vi "Initialize DAQ Assistant - Digital.vi"(8 "error in":errorcluster, 9 "rate":dbl=1000.0, 10 "number of samples":i32=100, 11 "physical channels":tag) -> (0 "error out":errorcluster, 3 "task out":refnum<k21>)   [LabVIEW 2021]
uses:
  <vilib>/DAQmx/create/channels.llb/DAQmx Create Channel (DI-Digital Input).vi
  <vilib>/DAQmx/configure/timing.llb/DAQmx Timing (Sample Clock).vi
  <resource>/objmgr/daqmx.rc
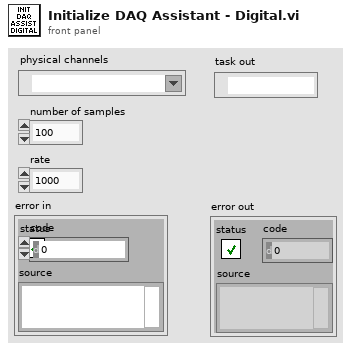
[diagram p1: front panel]
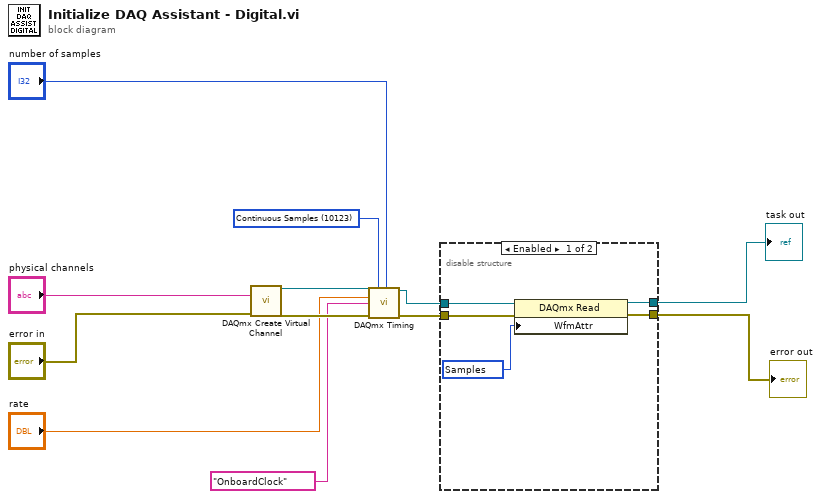
[diagram p0: block diagram]
diagram:
  w10 = 10123 items=["Finite Samples"=10178, "Continuous Samples"=10123, "Hardware Timed Single Point"=12522] ("sample mode")
  n1 = call-poly <vilib>:"DAQmx Create Virtual Channel.vi"("lines"="physical channels", "error in"="error in") -> ("task out"=w12:refnum<k21>, "error out"=w11:errorcluster)  [unwired: 12 in]
  n2 = call-poly <vilib>:"DAQmx Timing.vi"("task/channels in"=w12, "sample mode"=w10, "samples per channel"="number of samples", "rate"="rate", "source"=tag "OnboardClock", "error in"=w11) -> ("task out"=w5:refnum<k21>, "error out"=w4:errorcluster)  [unwired: 8 in]
  n3 = disable-structure shown="Enabled" {
    disable-tunnel: w5 -> [w16 w19]
    disable-tunnel: [w15 w19] -> w2
    disable-tunnel: w4 -> [w14 w18]
    disable-tunnel: [w13 w18] -> w1
    frame Enabled {
      w17 = 10287 items=["Samples"=10287, "Samples and Timing"=10140, "Samples, Timing, and Attributes"=10141] ("WfmAttr")
      n4 = property class="DAQmx Read"(reference=w16, error in=w14, "WfmAttr"=w17) -> (reference out=w15:refnum<k21>, error out=w13:errorcluster)
    }
    frame Disabled {
    }
  }
  "error out" <- w1
  "task out" <- w2
